vi "Kalman_Filter_Generator.vi"(8 "error in (no error)":errorcluster, 11 "Filter Constants":T1) -> (0 "error out":errorcluster, 3 "Kalman_Filter out":refnum<class "Kalman_Filter.lvclass">)   [LabVIEW 2021, in "Kalman_Filter.lvclass"]
uses:
  Kalman_Filter.lvclass
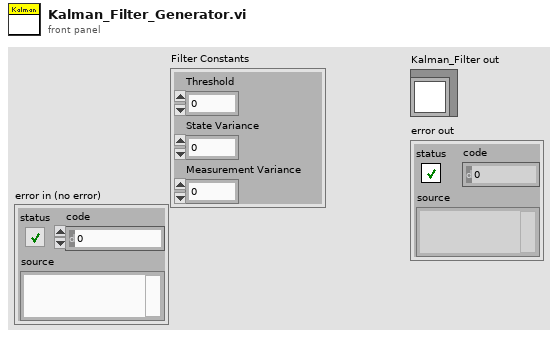
[diagram p1: front panel]
types:
  T1 = cluster{"Threshold":dbl, "State Variance":dbl, "Measurement Variance":dbl}
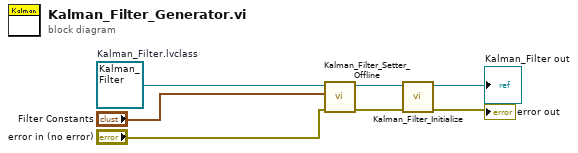
[diagram p0: block diagram]
diagram:
  w7 = refnum<class "Kalman_Filter.lvclass"> refnum  # Kalman_Filter.lvclass
  n1 = call-dynamic "Kalman_Filter_Setter_Offline.vi"("error in (no error)"="error in (no error)", "Filter Constants"="Filter Constants", "Kalman_Filter in"=w7) -> ("error out"=w6:errorcluster, "Kalman_Filter out"=w5:refnum<class "Kalman_Filter.lvclass">)  [unwired: 7 in]
  n2 = call-dynamic "Kalman_Filter_Initialize.vi"("error in (no error)"=w6, "Kalman_Filter in"=w5) -> ("error out"=→"error out":errorcluster, "Kalman_Filter out"=→"Kalman_Filter out":refnum<class "Kalman_Filter.lvclass">)  [unwired: 8 in]
